vi "Start.vi"() -> ()   [LabVIEW 2020]
uses:
  <vilib>/NI/Modbus Library/API/Wrapper/API Main.lvlib
  <vilib>/NI/Modbus Library/API/Wrapper/Create Serial Master.vi
  <vilib>/NI/Modbus Library/Transmission Data Unit/RTU/RTU Data Unit.lvclass
  <vilib>/NI/Modbus Library/API/Master/Modbus Master.lvclass
panel:
  out "string":string
  out "register values":u16[](array[numeric])
  in  "number of words":u16
  in  "starting address":u16
  in  "unit ID":u8=1
  in  "error in":errorcluster
  in  "VISA resource name":refnum<visa-resource-name>
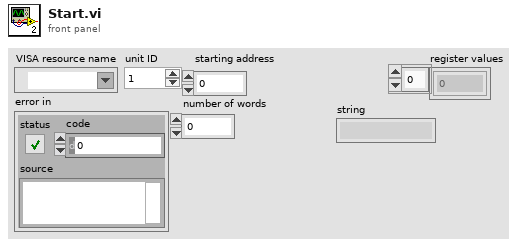
[diagram p1: front panel]
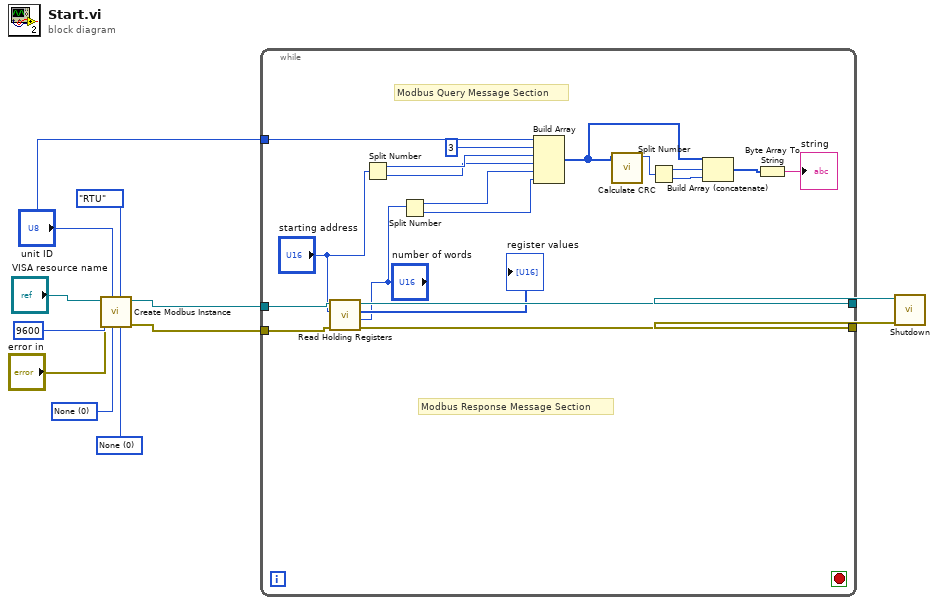
[diagram p0: block diagram]
diagram:
  w6 = u16 0 items=["None", "XON/XOFF", "RTS/CTS", "XON/XOFF & RTS/CTS", "DTR/DSR", "XON/XOFF & DTR/DSR"] ("flow control (none)")
  w7 = u16 0 items=["None", "Odd", "Even", "Mark", "Space"] ("parity (even)")
  n1 = call-poly <vilib>:"Create Modbus Instance.vi"("flow control (none)"=w6, "serial type"=enum16{"RTU", "ASCII"}."RTU", "parity (even)"=w7, "unit ID"="unit ID", "error in"="error in", "baud rate"=u32 9600, "VISA resource name"="VISA resource name") -> ("error out"=w4:errorcluster, "serial master instance"=w5:refnum<class "Modbus Master.lvclass">)  [unwired: 3 in]
  n2 = while {
    tunnel: w5 -> [w30]
    tunnel: w4 -> [w29]
    tunnel: [w28] -> w3
    tunnel: [w27] -> w2
    tunnel: "unit ID" -> [w25]
    stop <- _ stop-if-true
    # "Modbus Response Message Section"
    # "Modbus Query Message Section"
    n3 = call-dynamic "Read Holding Registers.vi"("error in"=w29, "number of inputs"="number of words", "starting address"="starting address", "Modbus master in"=w30) -> ("error out"=w27:errorcluster, "register values"=→"register values":u16[], "Modbus master out"=w28:refnum<class "Modbus Master.lvclass">)  [unwired: 5 in]
    n4 = Split Number(x="starting address") -> (hi(x)=w22:u8, lo(x)=w21:u8)
    n5 = Split Number(x="number of words") -> (hi(x)=w19:u8, lo(x)=w18:u8)
    n6 = Build Array(w25, u8 3 ("element"), w22, w21, w19, w18) -> (w14:u8[])
    n7 = call <vilib>:"Calculate CRC.vi"("data"=w14) -> ("CRC-16"=w17:u16)  [unwired: 10 in]
    n8 = Split Number(x=w17) -> (hi(x)=w16:u8, lo(x)=w15:u8)
    n9 = Build Array (concatenate)(w14, w16, w15) -> (w13:u8[])
    n10 = Byte Array To String(unsigned byte array=w13) -> (string=→"string":string)
  }
  n11 = call-dynamic "Shutdown.vi"("error in"=w2, "Modbus master in"=w3) -> ()  [unwired: 9 in, 1 out]
